vi "SetI2CFrequency.vi"(10 "I2C Frequency":enum8{"100kHz", "400kHz"}(ring)=enum."400kHz", 11 "Port":enum8{"ONE", "TWO"}(ring)) -> (3 "concatenated string":string)   [LabVIEW 2019]
panel:
  out "Checksum":u8=250 format="%x"
  out "Length":string
  out "Command ID":string
  out "SlaveID":string
  out "Data":string
  out "Port":string
  out "I2CFreq":string
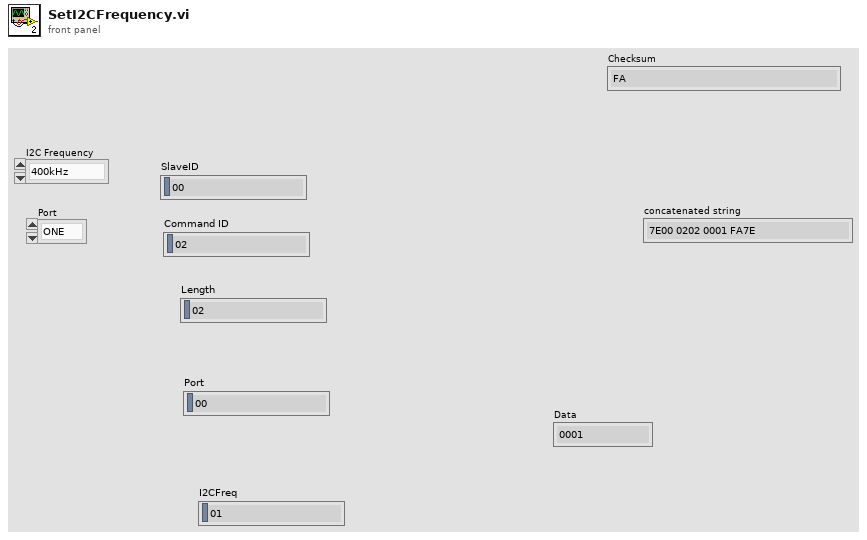
[diagram p1: front panel]
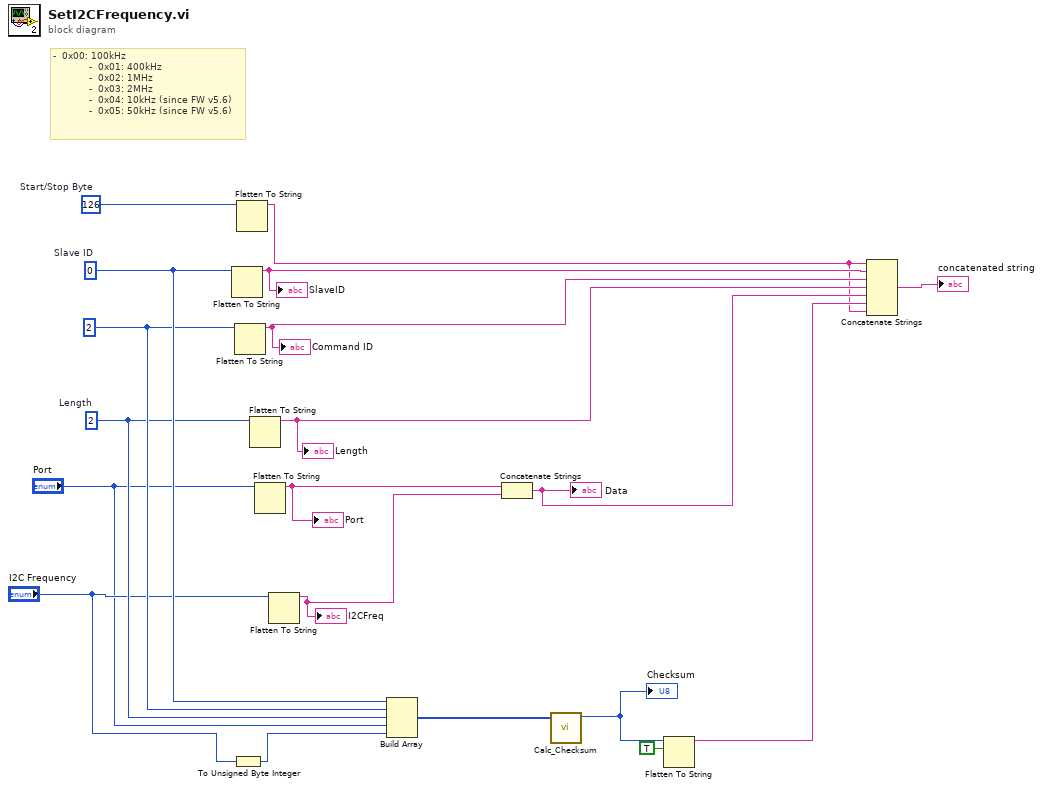
[diagram p0: block diagram]
diagram:
  w12 = u8 126  # Start/Stop Byte
  w11 = u8 0  # Slave ID
  w9 = u8 2  # Length
  w10 = u8 2 ("Command ID")
  # "-  0x00: 100kHz\n            -  0x01: 400kHz\n            -  0x02: 1MHz\n            -  0x03: 2MHz\n            -  0x04: 10kHz (since FW v5.6)\n            -  0x05: 50kHz (since FW v5.6)"
  n1 = Flatten To String(anything=w11) -> (data string=w17:string)  [unwired: 3 in, 2 out]
  "SlaveID" <- w17
  n2 = To Unsigned Byte Integer(number="I2C Frequency") -> (unsigned 8bit integer=w3:u8)
  n3 = Flatten To String(anything=w10) -> (data string=w16:string)  [unwired: 3 in, 2 out]
  "Command ID" <- w16
  n4 = Flatten To String(anything=w12) -> (data string=w5:string)  [unwired: 3 in, 2 out]
  n5 = Flatten To String(anything=w9) -> (data string=w15:string)  [unwired: 3 in, 2 out]
  "Length" <- w15
  n6 = Flatten To String(anything="Port") -> (data string=w18:string)  [unwired: 3 in, 2 out]
  "Port" <- w18
  n7 = Flatten To String(anything="I2C Frequency") -> (data string=w19:string)  [unwired: 3 in, 2 out]
  "I2CFreq" <- w19
  n8 = Build Array(w11, w10, w9, "Port", w3) -> (w8:u8[])
  n9 = Concatenate Strings(w18, w19) -> (w14:string)
  "Data" <- w14
  n10 = call "Calc_Checksum.vi"("DataFrame"=w8) -> ("Checksum"=w7:u8)  [unwired: 10 in]
  "Checksum" <- w7
  n11 = Flatten To String(anything=w7, prepend array or string size? (T)=TRUE) -> (data string=w6:string)  [unwired: 2 in, 2 out]
  n12 = Concatenate Strings(w5, w17, w16, w15, w14, w6, w5) -> (→"concatenated string":string)
